vi "Save config.vi"(8 "error in (no error)":errorcluster, 11 "DAQ Port":tag) -> (0 "error out":errorcluster)   [LabVIEW 2020]
uses:
  <vilib>/Utility/config.llb/NI_LVConfig.lvlib
  <vilib>/Utility/config.llb/Write Key (String).vi
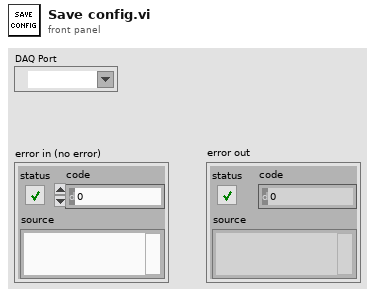
[diagram p1: front panel]
types:
  T1 = typedef "NI_LVConfig.lvlib/Config Data RefNum.ctl" = refnum<k1>
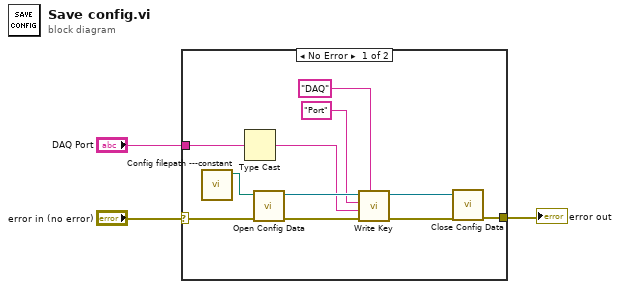
[diagram p0: block diagram]
diagram:
  n1 = case shown="No Error" "error in (no error)" {
    selector: "error in (no error)" -> [w13 w15]
    tunnel: [w7 w15] -> w2
    tunnel: "DAQ Port" -> [w5 _]
    frame No Error {
      n2 = call "Config filepath ---constant.vi"() -> ("config file path"=w14:path)  [unwired: 11 in]
      n3 = Type Cast(x=w5) -> (*(type *) &x=w4:string)  [unwired: 1 in]
      n4 = call <vilib>:"Open Config Data.vi"("error in (no error)"=w13, "configuration file path"=w14) -> ("error out"=w11:errorcluster, "refnum"=w12:T1)  [unwired: 7 in, 1 out]
      n5 = call-poly <vilib>:"Write Key.vi"("section"="DAQ", "error in (no error)"=w11, "value"=w4, "key"="Port", "refnum"=w12) -> ("error out"=w8:errorcluster, "refnum out"=w9:T1)  [unwired: 4 in, 1 out]
      n6 = call <vilib>:"Close Config Data.vi"("error in (no error)"=w8, "refnum"=w9) -> ("error out"=w7:errorcluster)  [unwired: 8 in, 1 out]
    }
    frame Error {
    }
  }
  "error out" <- w2
